vi "FABR-Initialize Level Axis.vi"(0 "XYGraph in":refnum<vi>, 5 "YAxis":refnum<vi>, 7 "Levels":dbl[](array[numeric]), 11 "error in (no error)":errorcluster) -> (15 "error out":errorcluster)   [LabVIEW 2020]
uses:
  epl-vi-lib/Utility VIs/Math VIs/LinSpace (x0-dx-npts).vi
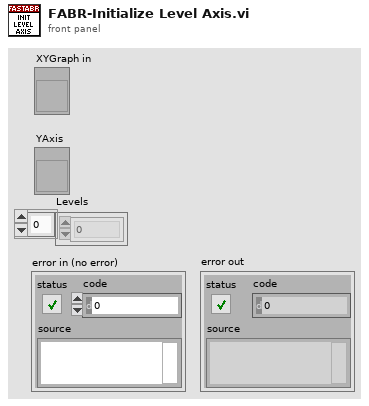
[diagram p1: front panel]
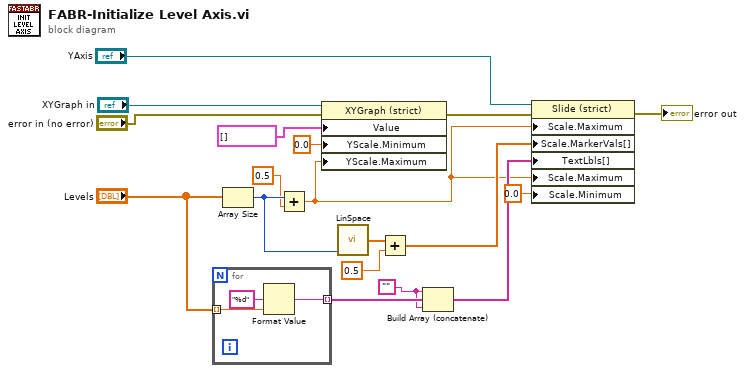
[diagram p0: block diagram]
diagram:
  w6 = ""
  n1 = for {
    tunnel: "Levels" -> [w21] mode=indexing
    tunnel: [w19] -> w9 mode=indexing
    n2 = Format Value(format string="%d", value (0)=w21) -> (output string=w19:string)  [unwired: 1 in]
  }
  n3 = Array Size(array="Levels") -> (size(s)=w3:i32)
  n4 = Add(x=w3, y=0.5) -> (x+y=w2:dbl)
  n5 = property class="XYGraph (strict)"(reference="XYGraph in", error in="error in (no error)", "Value"=cluster{dbl[], dbl[]}[] [], "YScale.Minimum"=0.0 ("X Scale.Range:Maximum"), "YScale.Maximum"=w2) -> (error out=w14:errorcluster)  [unwired: 1 out]
  n6 = call-poly "LinSpace.vi"("npts"=w3) -> ("Array"=w13:dbl[])  [unwired: 3 in, 1 out]
  n7 = Add(x=w13, y=0.5) -> (x+y=w11:dbl[])
  n8 = Build Array (concatenate)(w6, w9, w6) -> (w7:string[])
  n9 = property class="Slide (strict)"(reference="YAxis", error in=w14, "Scale.Maximum"=w2, "Scale.MarkerVals[]"=w11, "TextLbls[]"=w7, "Scale.Maximum"=w2, "Scale.Minimum"=0.0 ("Scale.Range:Minimum")) -> (error out=→"error out":errorcluster)  [unwired: 1 out]
